vi "WPI_DMAOpenInternal.vi"(8 "error in (no error)":errorcluster, 9 "Host Buffer Depth (Samples)":u32=512, 10 "Rate":dbl=1000.0) -> (0 "error out":errorcluster, 3 "DMARef":T1)   [LabVIEW 2017]
doc: "Opens a reference to the DMA stream from the FPGA of the roboRIO. You must open a reference before using any other VIs on this palette. You can have only one DMA stream open at a time. If you want to open a new DMA stream, use the Close VI to close the reference to the current DMA stream first.\n\nUses an internal sample clock to specify the frequency at which the FPGA sends data samples to the host buffer. Use this VI to specify the frequency.\n\nThis software is licensed. Open the labview\\readme\\WPI Robotics Library Open Source License.txt file for more information."
uses:
  <vilib>/Rock Robotics/WPI/DMA/WPI_DMARef.ctl
  <vilib>/Rock Robotics/SystemInterfaces/CounterEncoderSourceConvertion/FPGA_CounterEncoderSourceConvertionLVSourceType.ctl
  <vilib>/Rock Robotics/SystemInterfaces/DIO/FPGA_DIODigitalSourceChannel.ctl
  <vilib>/Rock Robotics/SystemInterfaces/AnalogTrigger/FPGA_AnalogTriggerIndex.ctl
  <vilib>/Rock Robotics/SystemInterfaces/AnalogTrigger/FPGA_AnalogTriggerOutType.ctl
  <vilib>/Rock Robotics/SystemInterfaces/DMA/FPGA_DMAWriteConfigOperation.ctl
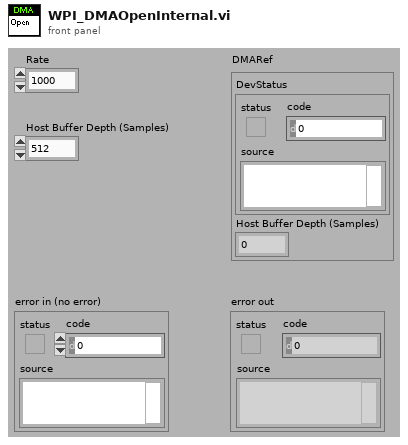
[diagram p1: front panel]
types:
  T1 = typedef "WPI_DMARef.ctl" = cluster{"DevStatus":errorcluster, "Host Buffer Depth (Samples)":u32}
  T2 = typedef "FPGA_CounterEncoderSourceConvertionLVSourceType.ctl" = cluster{"DevStatus":errorcluster, "AnalogTriggerMode?":bool, "DigitalMode":cluster{"DIO Channel":T3}, "AnalogTriggerMode":cluster{"AnalogTriggerIndex":T4, "OutputType":T5}}
  T3 = typedef "FPGA_DIODigitalSourceChannel.ctl" = enum8{"DIO 0", "DIO 1", "DIO 2", "DIO 3", "DIO 4", "DIO 5", "DIO 6", "DIO 7", "DIO 8", "DIO 9", "DIO MXP 0", "DIO MXP 1", "DIO MXP 2", "DIO MXP 3", "DIO MXP 4", "DIO MXP 5", "DIO MXP 6", "DIO MXP 7", "DIO MXP 8", "DIO MXP 9", "DIO MXP 10", "DIO MXP 11", "DIO MXP 12", "DIO MXP 13", "DIO MXP 14", "DIO MXP 15", "Disabled"}
  T4 = typedef "FPGA_AnalogTriggerIndex.ctl" = enum8{"Trig 0", "Trig 1", "Trig 2", "Trig 3", "Trig 4", "Trig 5", "Trig 6", "Trig 7", "Invalid"}
  T5 = typedef "FPGA_AnalogTriggerOutType.ctl" = enum16{"InWindow", "TriggerState", "Rising", "Falling"}
  T6 = cluster{"ExternalClock":bool, "ExternalTriggers":cluster{"DigitalSource":T2, "RisingEdge":bool, "FallingEdge":bool}[]}
  T7 = typedef "FPGA_DMAWriteConfigOperation.ctl" = enum16{"Update Pause", "Update Enable", "Update SampleClock"}
  T8 = typedef "WPI_DMAChannelTypeEnum.ctl" = enum16{"AI (Raw)", "AI (Avg)", "Accumulator", "DI (Raw) Onboard", "DI (Filtered) Onboard", "DI (Raw) MXP", "DI (Filtered) MXP", "Analog Trigger", "Counter", "Counter (Timer)", "Encoder", "Encoder (Timer)", "Time Stamp"}
  T9 = cluster{"Channel Type":T8, "Channel Number":u8}[]
  T10 = typedef "FPGA_DMADevRef.ctl" = cluster{"DevStatus":errorcluster}
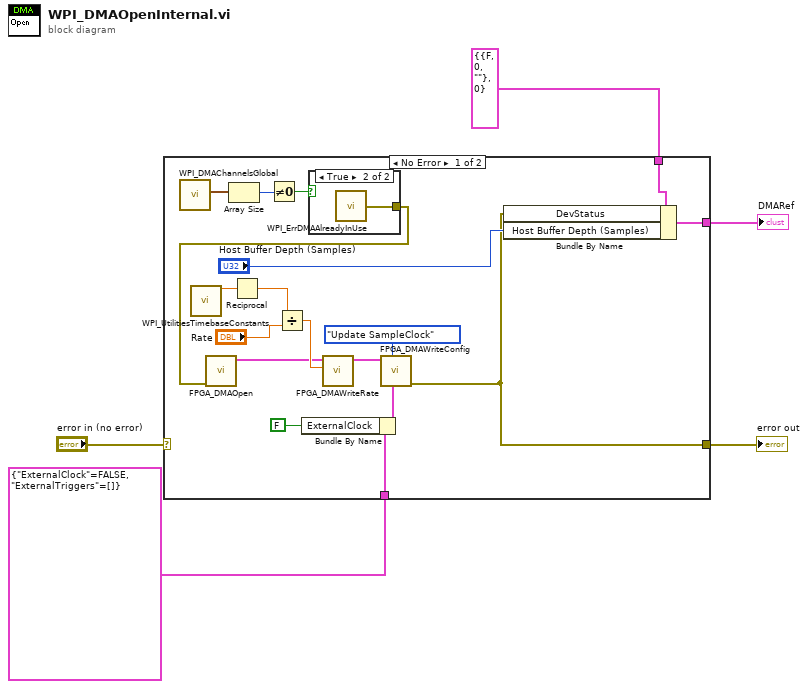
[diagram p0: block diagram]
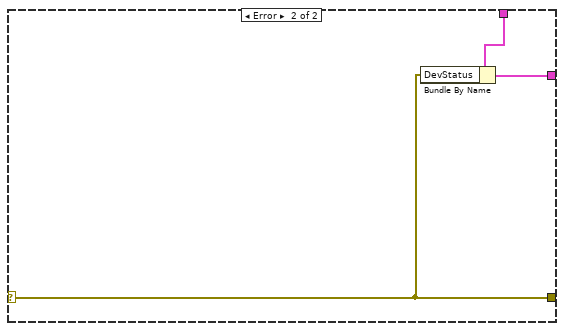
[diagram p3: hidden frame]
diagram:
  n1 = case shown="No Error" "error in (no error)" {
    selector: "error in (no error)" -> [_ w26]
    tunnel: [w9 w26] -> w4
    tunnel: [w22 w27] -> w3
    tunnel: T1 {"DevStatus"={"status"=FALSE, "code"=0, "source"=""}, "Host Buffer Depth (Samples)"=0} ("DMARef") -> [w23 w25]
    tunnel: T6 {"ExternalClock"=FALSE, "ExternalTriggers"=[]} ("SampleClock") -> [w11 _]
    frame No Error {
      n2 = call <vilib>:"WPI_DMAChannelsGlobal.vi"() -> ("Channels Out"=w16:T9)  [unwired: 4 in, 7 out]
      n3 = call <vilib>:"WPI_UtilitiesTimebaseConstants.vi"() -> ("40 MHz FPGA clock"=w7:dbl)  [unwired: 13 in, 2 out]
      n4 = Array Size(array=w16) -> (size(s)=w15:i32)
      n5 = Reciprocal(x=w7) -> (1/x=w6:dbl)
      n6 = Not Equal To 0?(x=w15) -> (x != 0?=w14:bool)
      n7 = Divide(x=w6, y="Rate") -> (x/y=w18:dbl)
      n8 = Bundle By Name(cluster=w11, "ExternalClock"=FALSE) -> (w8:T6)
      n9 = case shown="True" w14 {
        tunnel: [_ w24] -> w13
        frame False {
        }
        frame True {
          n10 = call <vilib>:"WPI_ErrDMAAlreadyInUse.vi"() -> ("error out"=w24:errorcluster)
        }
      }
      n11 = call <vilib>:"FPGA_DMAOpen.vi"("error in (no error)"=w13) -> ("DMADevRef"=w17:T10)  [unwired: 10 out]
      n12 = call <vilib>:"FPGA_DMAWriteRate.vi"("Rate"=w18, "DMADevRef In"=w17) -> ("DMADevRef Out"=w12:T10)  [unwired: 1 in, 8 out]
      n13 = call <vilib>:"FPGA_DMAWriteConfig.vi"("SampleClock"=w8, "Operation"=FPGA_DMAWriteConfigOperation."Update SampleClock", "DMADevRef"=w12) -> ("error out"=w9:errorcluster)  [unwired: 3 in, 5 out]
      n14 = Bundle By Name(cluster=w23, "DevStatus"=w9, "Host Buffer Depth (Samples)"="Host Buffer Depth (Samples)") -> (w22:T1)
    }
    frame Error {
      n15 = Bundle By Name(cluster=w25, "DevStatus"=w26) -> (w27:T1)
    }
  }
  "error out" <- w4
  "DMARef" <- w3
